vi "Update Steering Picture.vi"(5 "redraw grid (F)":bool, 7 "zoom to fit (F)":bool, 8 "error in (no error)":errorcluster, 11 "dialog info in":T1={"steering frame ref"=refnum, "active wheel indexes"=[], "FP Refs"={"VI Refnum"=refnum, "Menu Ref"=refnum, "Sub Panel"=refnum, "picture"=refnum, "Steering Type"=refnum, "zoom in"=refnum, "zoom out"=refnum, "zoom extents"=refnum, "Wheels"=refnum, "Add Wheel"=refnum, "Remove Wheel"=refnum, "Copy Wheel"=refnum, "Angle Units"=refnum}, "subpanel info"={"subpanel VI refs"=[], "subpanel types"=[], "main to subpanel command events"=[]}, "picture dragging state"={"dragging"=FALSE, "wheel index"=-1, "dragging mode"=enum."translate", "wheel start position"={"x"=0.0, "y"=0.0, "theta"=0.0}, "relative mouse position"={"x"=0.0, "y"=0.0}, "relative mouse init angle (rad)"=0.0}, "picture size (pixels)"={"Width"=500, "Height"=500}, "picture grid"=bytes[0], "click zones group"={"click zones array"=[], "num click zones"=0}, "draw options"={"draw wheel states?"=FALSE, "highlight wheel index"=-1, "pixels per unit"=10.0, "draw forward velocity?"=FALSE, "velocity scale"=1.0}}) -> (0 "error out":errorcluster, 3 "dialog info out":T1={"steering frame ref"=refnum, "active wheel indexes"=[], "FP Refs"={"VI Refnum"=refnum, "Menu Ref"=refnum, "Sub Panel"=refnum, "picture"=refnum, "Steering Type"=refnum, "zoom in"=refnum, "zoom out"=refnum, "zoom extents"=refnum, "Wheels"=refnum, "Add Wheel"=refnum, "Remove Wheel"=refnum, "Copy Wheel"=refnum, "Angle Units"=refnum}, "subpanel info"={"subpanel VI refs"=[], "subpanel types"=[], "main to subpanel command events"=[]}, "picture dragging state"={"dragging"=FALSE, "wheel index"=-1, "dragging mode"=enum."translate", "wheel start position"={"x"=0.0, "y"=0.0, "theta"=0.0}, "relative mouse position"={"x"=0.0, "y"=0.0}, "relative mouse init angle (rad)"=0.0}, "picture size (pixels)"={"Width"=500, "Height"=500}, "picture grid"=bytes[0], "click zones group"={"click zones array"=[], "num click zones"=0}, "draw options"={"draw wheel states?"=FALSE, "highlight wheel index"=-1, "pixels per unit"=10.0, "draw forward velocity?"=FALSE, "velocity scale"=1.0}})   [LabVIEW 2017, in "NI_Robotics_Configure Steering Frame.lvlib"]
uses:
  <vilib>/robotics/Dialog/Configure Steering Frame/NI_Robotics_Configure Steering Frame.lvlib
  <vilib>/robotics/Dialog/Configure Steering Frame/Dialog Info.ctl
  <vilib>/robotics/Steering/Steering Frame/NI_Robotics_Steering Frame.lvclass
  <vilib>/robotics/Dialog/Configure Steering Frame/FP Refs.ctl
  <vilib>/robotics/Dialog/Configure Steering Frame/Subpanel Info.ctl
  <vilib>/robotics/Dialog/Configure Steering Frame/Main to Subpanel Command Event.ctl
  <vilib>/robotics/Dialog/Configure Steering Frame/Main to Subpanel Command.ctl
  <vilib>/robotics/Dialog/Configure Steering Frame/Dragging State.ctl
  <vilib>/robotics/Dialog/Configure Steering Frame/Dragging Mode.ctl
  <vilib>/Utility/miscctls.llb/LVBoundsTypeDef.ctl
  <vilib>/robotics/Dialog/Configure Steering Frame/Click Zone.ctl
  <vilib>/robotics/Utilities/Visualization/Steering Visualization/Steering Picture/Draw Steering Frame Options.ctl
  <vilib>/robotics/Steering/Steering Frame/NI_Robotics_Steering Frame.lvclass/NI_Robotics_Steering Frame.ctl
  <vilib>/robotics/Steering/Wheel/NI_Robotics_Wheel.lvclass/NI_Robotics_Wheel.ctl
  <vilib>/robotics/Dialog/Configure Steering Frame/Get Steering Frame Bounds.vi
  <vilib>/robotics/Dialog/Configure Steering Frame/Coerce Pixels per Unit.vi
  <vilib>/robotics/Steering/Steering Frame/Get Wheels in Steering Frame.vi
  <vilib>/robotics/Steering/Steering Frame/Get Multiple Wheels in Steering Frame.vi
  <vilib>/robotics/Steering/Wheel/Get Wheel Radius.vi
  <vilib>/robotics/Steering/Wheel/NI_Robotics_Wheel.lvclass
  <vilib>/robotics/Utilities/Visualization/Steering Visualization/Steering Picture/NI_Robotics_Steering Picture.lvlib
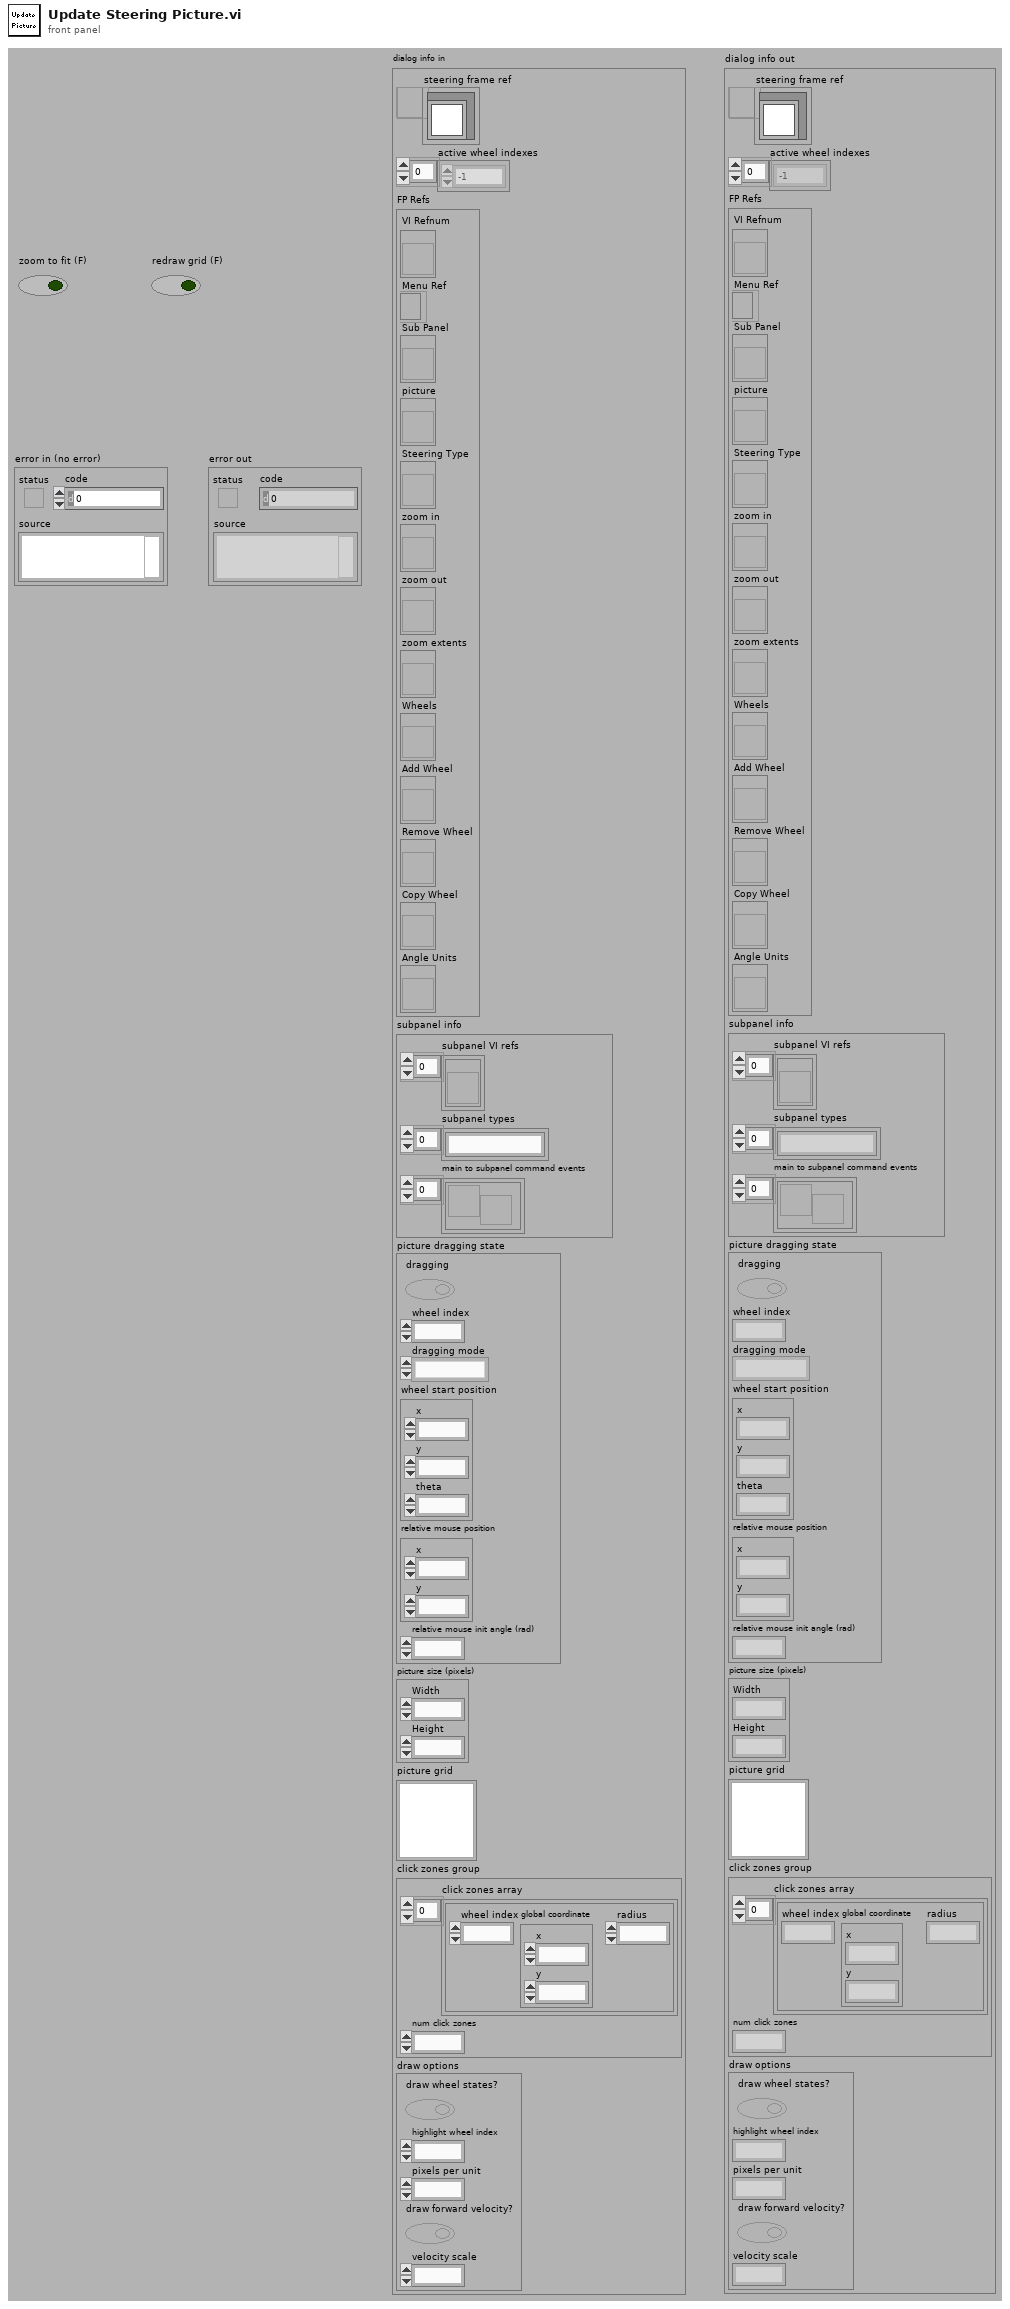
[diagram p1: front panel]
types:
  T1 = typedef "NI_Robotics_Configure Steering Frame.lvlib/Dialog Info.ctl" = cluster{"steering frame ref":refnum<data-value>, "active wheel indexes":i32[], "FP Refs":T2, "subpanel info":T3, "picture dragging state":T5, "picture size (pixels)":T7, "picture grid":picture, "click zones group":cluster{"click zones array":T8[], "num click zones":i32}, "draw options":T9}
  T2 = typedef "NI_Robotics_Configure Steering Frame.lvlib/FP Refs.ctl" = cluster{"VI Refnum":refnum<vi>, "Menu Ref":refnum<k9>, "Sub Panel":refnum<vi>, "picture":refnum<vi>, "Steering Type":refnum<vi>, "zoom in":refnum<vi>, "zoom out":refnum<vi>, "zoom extents":refnum<vi>, "Wheels":refnum<vi>, "Add Wheel":refnum<vi>, "Remove Wheel":refnum<vi>, "Copy Wheel":refnum<vi>, "Angle Units":refnum<vi>}
  T3 = typedef "NI_Robotics_Configure Steering Frame.lvlib/Subpanel Info.ctl" = cluster{"subpanel VI refs":refnum<vi>[], "subpanel types":string[], "main to subpanel command events":T4[]}
  T4 = typedef "NI_Robotics_Configure Steering Frame.lvlib/Main to Subpanel Command Event.ctl" = refnum<user-event>
  T5 = typedef "NI_Robotics_Configure Steering Frame.lvlib/Dragging State.ctl" = cluster{"dragging":bool, "wheel index":i32, "dragging mode":T6, "wheel start position":cluster{"x":dbl, "y":dbl, "theta":dbl}, "relative mouse position":cluster{"x":dbl, "y":dbl}, "relative mouse init angle (rad)":dbl}
  T6 = typedef "NI_Robotics_Configure Steering Frame.lvlib/Dragging Mode.ctl" = enum16{"translate", "rotate"}
  T7 = typedef "LVBoundsTypeDef.ctl" = cluster{"Width":u32, "Height":u32}
  T8 = typedef "NI_Robotics_Configure Steering Frame.lvlib/Click Zone.ctl" = cluster{"wheel index":i32, "global coordinate":cluster{"x":dbl, "y":dbl}, "radius":dbl}
  T9 = typedef "NI_Robotics_Steering Picture.lvlib/Draw Steering Frame Options.ctl" = cluster{"draw wheel states?":bool, "highlight wheel index":i32, "pixels per unit":dbl, "draw forward velocity?":bool, "velocity scale":dbl}
  T10 = cluster{"click zones array":T8[], "num click zones":i32}
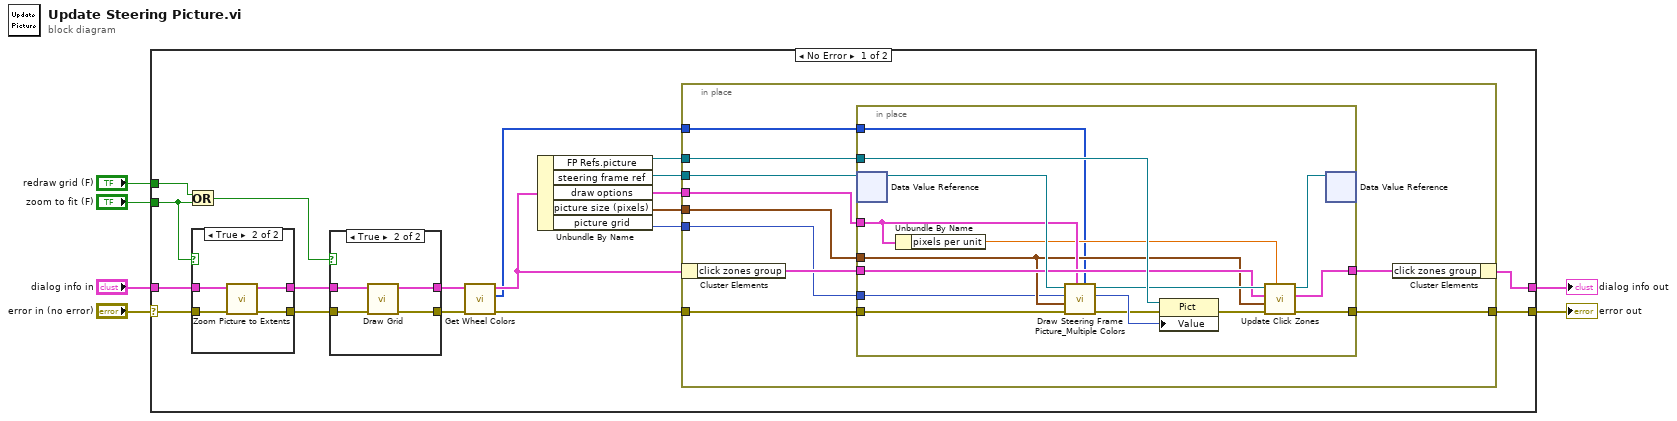
[diagram p0: block diagram]
diagram:
  n1 = case shown="No Error" "error in (no error)" {
    selector: "error in (no error)" -> [w23 w65]
    tunnel: "dialog info in" -> [w22 w64]
    tunnel: [w25 w65] -> w4
    tunnel: [w24 w64] -> w3
    tunnel: "zoom to fit (F)" -> [w13 _]
    tunnel: "redraw grid (F)" -> [w14 _]
    frame No Error {
      n2 = Or(x=w14, y=w13) -> (x .or. y?=w12:bool)
      n3 = case shown="True" w13 {
        tunnel: w23 -> [w33 w37]
        tunnel: [w33 w36] -> w15
        tunnel: w22 -> [w32 w35]
        tunnel: [w32 w34] -> w16
        frame False {
        }
        frame True {
          n4 = call <vilib>:"Zoom Picture to Extents.vi"("error in (no error)"=w37, "dialog info in"=w35) -> ("error out"=w36:errorcluster, "dialog info out"=w34:T1)  [unwired: 8 in]
        }
      }
      n5 = case shown="True" w12 {
        tunnel: w16 -> [w27 w29]
        tunnel: [w27 w28] -> w9
        tunnel: w15 -> [w26 w31]
        tunnel: [w26 w30] -> w11
        frame False {
        }
        frame True {
          n6 = call <vilib>:"Draw Grid.vi"("error in (no error)"=w31, "dialog info in"=w29) -> ("error out"=w30:errorcluster, "dialog info out"=w28:T1)  [unwired: 8 in]
        }
      }
      n7 = call <vilib>:"Get Wheel Colors.vi"("error in (no error)"=w11, "dialog info in"=w9) -> ("error out"=w10:errorcluster, "wheel colors"=w7:u32[], "dialog info out"=w8:T1)  [unwired: 7 in]
      n8 = Unbundle By Name(w8) -> ("FP Refs.picture"=w21:refnum<vi>, "steering frame ref"=w20:refnum<data-value>, "draw options"=w19:T9, "picture size (pixels)"=w18:T7, "picture grid"=w17:picture)
      n9 = in-place {
        in-place-border: w10 -> [w47]
        in-place-border: [w46] -> w25
        in-place-border: w21 -> [w43]
        in-place-border: w20 -> [w42]
        in-place-border: w19 -> [w41]
        in-place-border: w18 -> [w40]
        in-place-border: w17 -> [w39]
        in-place-border: w7 -> [w38]
        n10 = in-place-cluster #1(w8) -> ("click zones group"=w45:T10)
        n11 = in-place {
          in-place-border: w47 -> [w50]
          in-place-border: [w58] -> w46
          in-place-border: w43 -> [w63]
          in-place-border: w41 -> [w53]
          in-place-border: w40 -> [w52]
          in-place-border: w45 -> [w55]
          in-place-border: [w54] -> w44
          in-place-border: w39 -> [w49]
          in-place-border: w38 -> [w48]
          n12 = in-place-dvr #2(w42) -> (w62:refnum<class "NI_Robotics_Steering Frame.lvclass">)  [unwired: 1 out]
          n13 = Unbundle By Name(w53) -> ("pixels per unit"=w51:dbl)
          n14 = call <vilib>:"Draw Steering Frame Picture_Multiple Colors.vi"("wheel colors"=w48, "drawing options"=w53, "error in (no error)"=w50, "picture draw area size (pixels)"=w52, "picture in"=w49, "steering frame in"=w62) -> ("error out"=w60:errorcluster, "picture out"=w61:picture, "steering frame out"=w57:refnum<class "NI_Robotics_Steering Frame.lvclass">)  [unwired: 3 in]
          n15 = property class="Pict"(reference=w63, error in=w60, "Value"=w61) -> (error out=w59:errorcluster)  [unwired: 1 out]
          n16 = call <vilib>:"Update Click Zones.vi"("pixels per unit"=w51, "error in (no error)"=w59, "picture size (pixels)"=w52, "click zones group in"=w55, "steering frame in"=w57) -> ("error out"=w58:errorcluster, "click zones group out"=w54:T10, "steering frame out"=w56:refnum<class "NI_Robotics_Steering Frame.lvclass">)  [unwired: 4 in]
          n17 = in-place-dvr #2(w56) -> ()  [unwired: 2 out]
        }
        n18 = in-place-cluster #1("click zones group"=w44) -> (w24:T1)
      }
    }
    frame Error {
    }
  }
  "dialog info out" <- w3
  "error out" <- w4
